vi "getTimerResolution.vi"(8 "error in (no error)":errorcluster, 11 "CCD in":refnum<class "CCD.lvclass">) -> (0 "error out":errorcluster, 1 "resolution [us]":i32, 2 "resolution":T1=enum."1 - Sets the timer resolution to 1 microsecond", 3 "CCD out":refnum<class "CCD.lvclass">)   [LabVIEW 2023, in "CCD.lvclass"]
uses:
  CCD.lvclass
  TimerResolutionEnum.ctl
  TimerResolution.ctl
  20f7d3bd-08ac-4524-9bed-df36c1da25a0.vi
  a21955fc-e3a0-4e36-8495-41f1bfac7860.vi
  <vilib>/JDP Science/JSONtext/Variant to JSON Text.vi
  <vilib>/JDP Science/JSONtext/Set Item.vi
  <vilib>/JDP Science/JSONtext/JSON text to Variant.vi
  <vilib>/JDP Science/JSONtext/LVClass Serializer/JSONtext LVClass Serializer.lvclass
  CCD.lvclass/CCD.ctl
  GenericDevice/GenericDevice.lvclass
  <vilib>/IlluminatedG/lv-web-crypto/lv-json/JSON/JSON.lvlib
panel:
  # "Connector Pane"
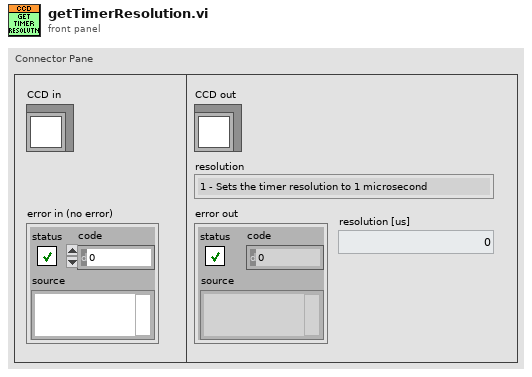
[diagram p1: front panel]
types:
  T1 = typedef "CCD.lvclass/TimerResolutionEnum.ctl" = enum16{"0 - Sets the timer resolution to 1000 microseconds", "1 - Sets the timer resolution to 1 microsecond"}
  T2 = typedef "CCD.lvclass/TimerResolution.ctl" = cluster{"resolution":i32}
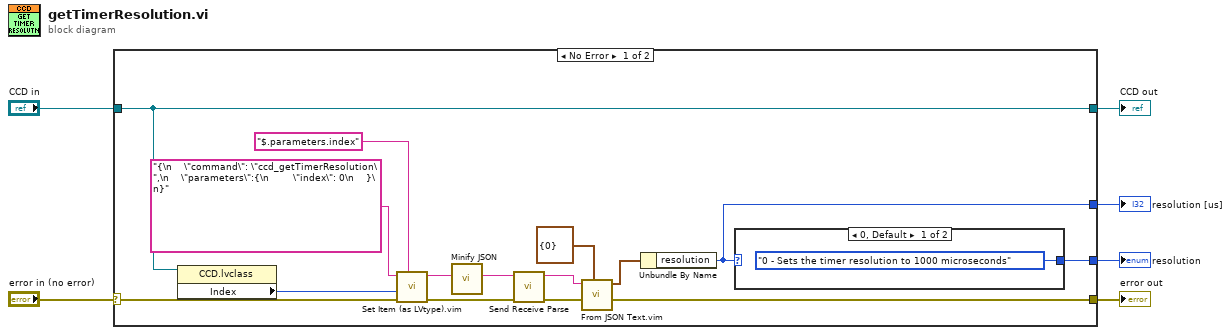
[diagram p0: block diagram]
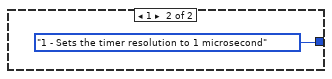
[diagram p2: hidden frame]
diagram:
  n1 = case shown="No Error" "error in (no error)" {
    selector: "error in (no error)" -> [w17 w25]
    tunnel: [w16 w25] -> w5
    tunnel: [w19 w24] -> w3
    tunnel: "CCD in" -> [w19 w24]
    tunnel: [w8 _] -> w2
    tunnel: [w7 _] -> w1
    frame No Error {
      n2 = property class="CCD.lvclass"(reference=w19) -> ("Index"=w18:i32)  [unwired: 1 in, 2 out]
      n3 = call "Set Item (as LVtype).vim"("$Path or Item Name"="$.parameters.index", "error in (no error)"=w17, "Anything"=w18, "JSON"="{\n    \"command\": \"ccd_getTimerResolution\",\n    \"parameters\":{\n        \"index\": 0\n    }\n}") -> ("error out"=w14:errorcluster, "<JSON>"=w10:string)  [unwired: 4 in, 1 out]
      n4 = call <vilib>:"Minify JSON.vi"("JSON String"=w10) -> ("Minified JSON"=w9:string)  [unwired: 10 in]
      n5 = call "Send Receive Parse.vi"("error in"=w14, "<JSON>"=w9) -> ("error out"=w13:errorcluster, "results-JSON string"=w15:string)  [unwired: 7 in, 1 out]
      n6 = call "From JSON Text.vim"("Data Type and Default Value"=T2 {"resolution"=0} ("exposure time"), "error in (no error)"=w13, "JSON"=w15) -> ("error out"=w16:errorcluster, "Data out"=w11:T2)  [unwired: 7 in]
      n7 = Unbundle By Name(w11) -> ("resolution"=w7:i32)
      n8 = case shown="0, Default" w7 {
        tunnel: [TimerResolutionEnum."0 - Sets the timer resolution to 1000 microseconds" ("resolution") TimerResolutionEnum."1 - Sets the timer resolution to 1 microsecond" ("resolution")] -> w8
        frame 0, Default {
        }
        frame 1 {
        }
      }
    }
    frame Error {
    }
  }
  "error out" <- w5
  "CCD out" <- w3
  "resolution" <- w2
  "resolution [us]" <- w1
